vi "Instrument Reset.vi"(8 "error in":errorcluster, 10 "Reset?":bool, 11 "AcopianERP in":refnum<class "Acopian.lvclass">) -> (0 "error out":errorcluster, 3 "AcopianERP out":refnum<class "Acopian.lvclass">)   [LabVIEW 2019, in "Acopian.lvlib" / "Acopian.lvclass"]
uses:
  Library/Acopian.lvclass
  Library/Acopian.lvclass/Acopian.ctl
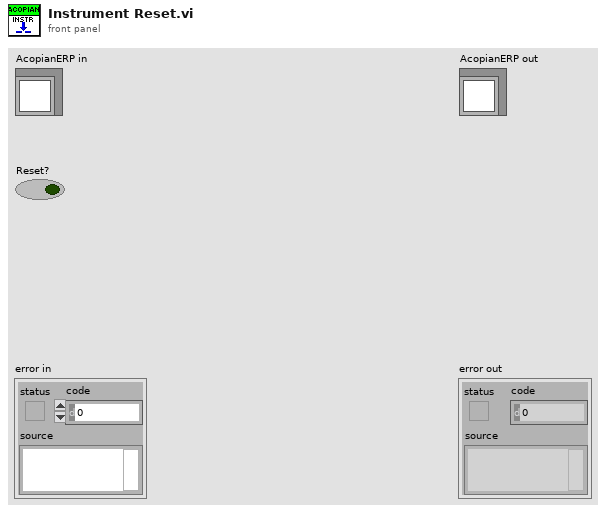
[diagram p1: front panel]
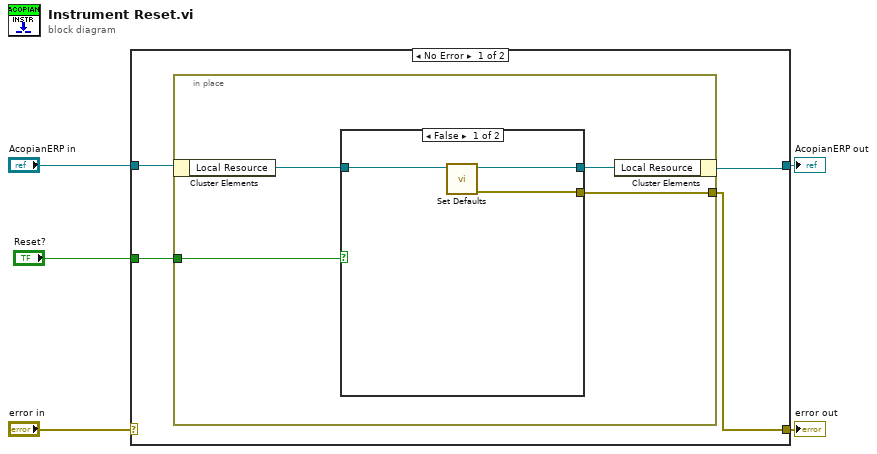
[diagram p0: block diagram]
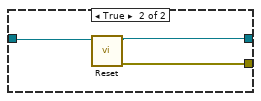
[diagram p2: hidden frame]
diagram:
  n1 = case shown="No Error" "error in" {
    selector: "error in" -> [_ w21]
    tunnel: [w8 w21] -> w4
    tunnel: [w6 w20] -> w2
    tunnel: "AcopianERP in" -> [w9 w20]
    tunnel: "Reset?" -> [w7 _]
    frame No Error {
      n2 = in-place {
        in-place-border: [w11] -> w8
        in-place-border: w7 -> [w10]
        n3 = in-place-cluster #1(w9) -> ("Local Resource"=w13:refnum<visa-resource-name>)
        n4 = case shown="False" w10 {
          tunnel: w13 -> [w16 w19]
          tunnel: [w15 w18] -> w12
          tunnel: [w14 w17] -> w11
          frame False {
            n5 = call "Set Defaults.vi"("VISA resource name"=w16) -> ("error out"=w14:errorcluster, "VISA resource name out"=w15:refnum<visa-resource-name>)  [unwired: 9 in]
          }
          frame True {
            n6 = call "Reset.vi"("VISA resource name"=w19) -> ("error out"=w17:errorcluster, "VISA resource out"=w18:refnum<visa-resource-name>)  [unwired: 9 in]
          }
        }
        n7 = in-place-cluster #1("Local Resource"=w12) -> (w6:refnum<class "Acopian.lvclass">)
      }
    }
    frame Error {
    }
  }
  "error out" <- w4
  "AcopianERP out" <- w2
